vi "Read (No Check).vi"   [LabVIEW 2016, in "Memory Manager.lvlib" / "Pointer.lvclass"]
doc: "Reads the contents of <b>pointer</b> into <b>value</b>."
uses:
  Pointer.lvclass
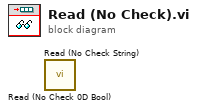
[diagram p0: block diagram]
diagram:
  n1 = call "Read (No Check 0D Bool).vi"() -> ()  [unwired: 8 in, 4 out]
  n2 = call "Read (No Check String).vi"() -> ()  [unwired: 8 in, 4 out]
